vi "HIOKI PW3390 Measure.vi"(0 "VISA Resource":refnum<visa-resource-name>, 5 "Item":T1(array[cluster]), 11 "error in (no error)":errorcluster, 13 "Error Out (F: Off)":bool) -> (3 "Status out":string, 4 "VISA Resource out":refnum<visa-resource-name>, 6 "Selected Item out":string[](array[string]), 8 "Data out":dbl[](array[numeric]), 10 "String out":string[](array[string]), 15 "error out":errorcluster)   [LabVIEW 2018]
doc: "Reads the measurement data.\n\n<B>Note</B>\nWhen the item number is more than 0\n Creates measurement data specified by the Item. Up to a maximum of 64 items. Items are arranged arbitrarily, and data is created in the order specified.\n Ch configuration of the Item after CH A is unnecessary.\n\nWhen the item number is 0\n Creates measurement data specified by \"HIOKI PW3390 Conf Measure Item.vi\". In this case, the measurement data's order is fixed. (Refer to output items and order)\n\nSelected Item out\n Returns the measurement item.\n\nData out\n Returns the measurement data.\nString out\n Returns the measurement data as string."
panel:
  # "Item(0: U)"
  # "Ch(0:Ch1)"
  # "Item0"
  # "Item1"
  # "Item2"
  # "Item3"
  # "Item4"
  # "Item5"
  # "Item6"
  # "Item7"
  # "Item8"
  # "Item9"
  # "Item10"
  # "Item11"
  # "Item12"
  # "Item13"
  # "Item14"
  # "Item15"
  # ":"
  # "Item63"
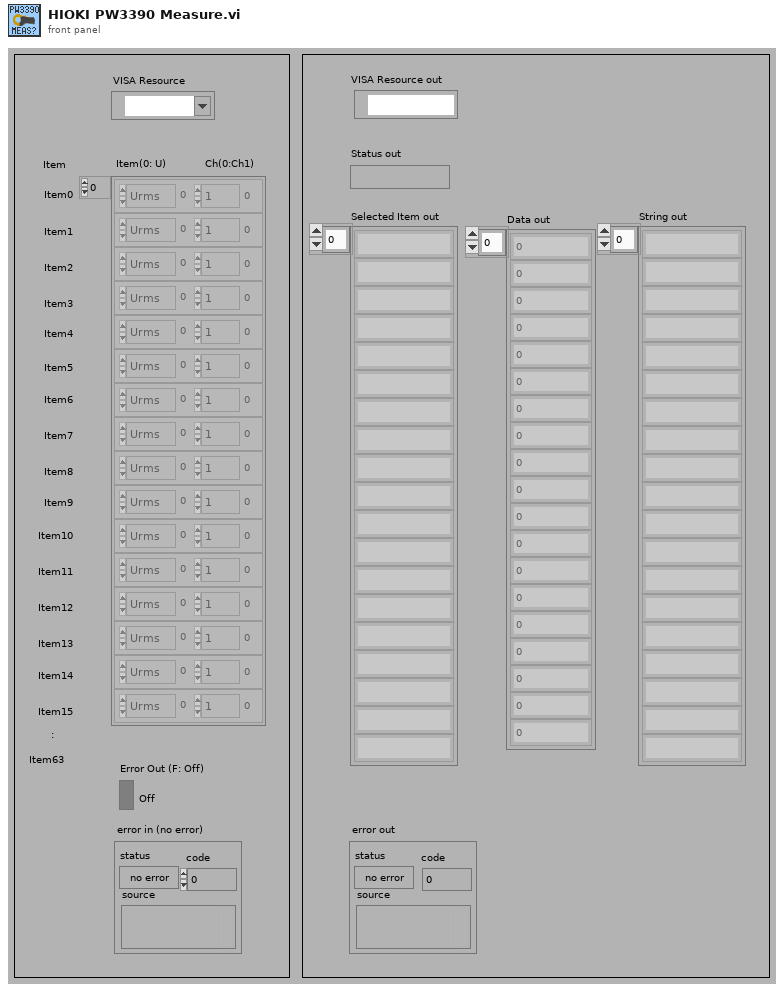
[diagram p1: front panel]
types:
  T1 = cluster{"Item":enum16{"Urms", "Umn", "Uac", "Udc", "Ufnd", "Upk+", "Upk-", "Uthd", "Urf", "Uunb", "Irms", "Imn", "Iac", "Idc", "Ifnd", "Ipk+", "Ipk-", "Ithd", "Irf", "Iunb", "P", "S", "Q", "PF", "DEG U", "DEG I", "DEG P", "f", "EFFI", "LOSS", "IH+", "IH-", "IH", "WP+", "WP-", "WP", "CH A", "CH B", "Pm", "Slip", "Laptime", "Laptime(ms)"}, "Ch(0:Ch1)":enum16{"1", "2", "3", "4", "12", "34", "123"}}[]
  T2 = enum16{"Urms", "Umn", "Uac", "Udc", "Ufnd", "Upk+", "Upk-", "Uthd", "Urf", "Uunb", "Irms", "Imn", "Iac", "Idc", "Ifnd", "Ipk+", "Ipk-", "Ithd", "Irf", "Iunb", "P", "S", "Q", "PF", "DEG U", "DEG I", "DEG P", "f", "EFFI", "LOSS", "IH+", "IH-", "IH", "WP+", "WP-", "WP", "CH A", "CH B", "Pm", "Slip", "Laptime", "Laptime(ms)"}
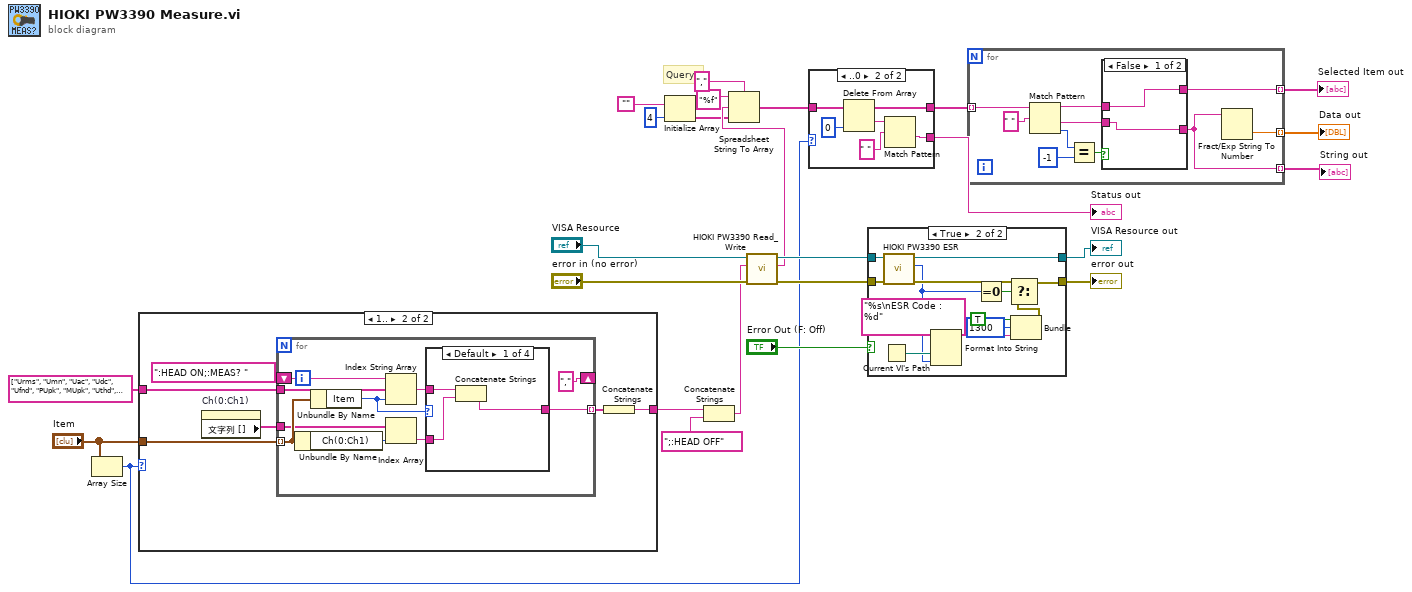
[diagram p0: block diagram]
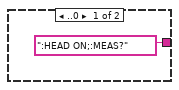
[diagram p4: hidden frame]
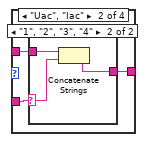
[diagram p5: hidden frame]
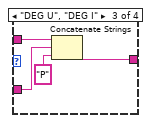
[diagram p7: hidden frame]
diagram:
  # "Query"
  n1 = Array Size(array="Item") -> (size(s)=w6:i32)
  n2 = case shown="1.." w6 {
    tunnel: "Item" -> [_ w28]
    tunnel: [":HEAD ON;:MEAS?" w32] -> w9
    tunnel: string[] ["Urms", "Umn", "Uac", "Udc", "Ufnd", "PUpk", "MUpk", "Uthd", "Urf", "Uunb", "Irms", "Imn", "Iac", "Idc", "Ifnd", "PIpk", "MIpk", "Ithd", "Irf", "Iunb", "P", "S", "Q", "PF", "HU", "HI", "DEG", "FREQ", "Eff", "Loss", "PIH", "MIH", "IH", "PWP", "MWP", "WP", "ExtA", "ExtB", "Pm", "Slip", "Laptime", "Laptime(ms)"] ("Strings []") -> [_ w30]
    frame ..0 {
    }
    frame 1.. {
      n3 = property on="Ch(0:Ch1)" class="Enum (strict)"() -> ("文字列 []"=w29:string[])  [unwired: 2 in, 2 out]
      n4 = for {
        shift-right: [","] -> _
        shift-left: ":HEAD ON;:MEAS? " -> [w42]
        tunnel: [w34] -> w27 mode=indexing
        tunnel: w28 -> [w40] mode=indexing
        tunnel: w30 -> [w39]
        tunnel: w29 -> [w38]
        n5 = Unbundle By Name(w40) -> ("Ch(0:Ch1)"=w33:enum16{"1", "2", "3", "4", "12", "34", "123"})
        n6 = Unbundle By Name(w40) -> ("Item"=w35:T2)
        n7 = Index String Array(1:w35, 2:w39, 3:w42) -> (0:w37:string)
        n8 = Index Array(array=w38, index=w33) -> (element=w36:string)
        n9 = case shown="Default" w35 {
          tunnel: w37 -> [w45 w48 w56 w57]
          tunnel: w36 -> [w44 w46 w55 _]
          tunnel: [w43 w47 w54 w57] -> w34
          frame Default {
            n10 = Concatenate Strings(w45, w44) -> (w43:string)
          }
          frame "Uac", "Iac" {
            n11 = case shown="\"1\", \"2\", \"3\", \"4\"" w46 {
              selector: w46 -> [_ w50]
              tunnel: w48 -> [w49 w52]
              tunnel: [w49 w51] -> w47
              frame Default {
              }
              frame "1", "2", "3", "4" {
                n12 = Concatenate Strings(w52, w50) -> (w51:string)
              }
            }
          }
          frame "DEG U", "DEG I" {
            n13 = Concatenate Strings(w56, w55, "P" ("文字列")) -> (w54:string)
          }
          frame "CH A".. {
          }
        }
      }
      n14 = Concatenate Strings(w27) -> (w32:string)
    }
  }
  n15 = Initialize Array("", 4) -> (w16:string[])
  n16 = Concatenate Strings(w9, ";:HEAD OFF") -> (w7:string)
  n17 = call "HIOKI PW3390 Read_Write.vi"("error in (no error)"="error in (no error)", "data in"=w7, "VISA Resource"="VISA Resource") -> ("error out"=w23:errorcluster, "data out"=w20:string, "VISA Resource out"=w24:refnum<visa-resource-name>)  [unwired: 6 in]
  n18 = Spreadsheet String To Array(delimiter (Tab)=",", format string="%f", spreadsheet string=w20, array type (2D Dbl)=w16) -> (array=w5:string[])
  n19 = case shown="..0" w6 {
    tunnel: w5 -> [w58 w64]
    tunnel: [w58 w62] -> w4
    tunnel: [_ w59] -> w12
    frame 1.. {
    }
    frame ..0 {
      n20 = Delete From Array(array=w64, index=0 ("指標")) -> (deleted portion=w61:string, array with subset deleted=w62:string[])  [unwired: 1 in]
      n21 = Match Pattern(string=w61, regular expression=" ") -> (after substring=w59:string)  [unwired: 1 in, 3 out]
    }
  }
  "Status out" <- w12
  n22 = case shown="True" "Error Out (F: Off)" {
    tunnel: w24 -> [w66 w79]
    tunnel: w23 -> [w65 w78]
    tunnel: [w65 w68] -> w22
    tunnel: [w66 w77] -> w10
    frame False {
    }
    frame True {
      n23 = Current VI's Path() -> (path=w75:path)
      n24 = call "HIOKI PW3390 ESR.vi"("error in (no error)"=w78, "VISA Resource"=w79) -> ("error out"=w69:errorcluster, "Output Value"=w67:u8, "VISA Resource out"=w77:refnum<visa-resource-name>)  [unwired: 6 in, 1 out]
      n25 = Format Into String(format string="%s\nESR Code : %d", w75, w67) -> (resulting string=w71:string)  [unwired: 2 in, 1 out]
      n26 = Equal To 0?(x=w67) -> (x = 0?=w76:bool)
      n27 = Bundle("status"=TRUE, "code"=1300, w71) -> (w70:cluster{"status":bool, "code":i32, string})  [unwired: 1 in]
      n28 = Select(t=w69, s=w76, f=w70) -> (s? t:f=w68:errorcluster)
    }
  }
  "error out" <- w22
  "VISA Resource out" <- w10
  n29 = for {
    tunnel: w4 -> [w89] mode=indexing
    tunnel: [w87] -> w3 mode=indexing
    tunnel: [w80] -> w2 mode=indexing
    tunnel: [w81] -> w1 mode=indexing
    n30 = Match Pattern(string=w89, regular expression=" ") -> (before substring=w83:string, after substring=w82:string, offset past match=w86:i32)  [unwired: 1 in, 1 out]
    n31 = Equal?(x=w86, y=-1 ("x")) -> (x = y?=w84:bool)
    n32 = case shown="False" w84 {
      tunnel: w83 -> [w91 w92]
      tunnel: w82 -> [w90 _]
      tunnel: [w90 w92] -> w81
      tunnel: [w91 _] -> w80
      frame False {
      }
      frame True {
      }
    }
    n33 = Fract/Exp String To Number(string=w81) -> (number=w87:dbl)  [unwired: 3 in, 1 out]
  }
  "Data out" <- w3
  "Selected Item out" <- w2
  "String out" <- w1
